vi "CRYMessage Dialog.vi"(7 "Window Title":string, 10 "YesNoCancel":T1(ring), 11 "Message Content":string) -> (2 "YesNo":bool=TRUE, 3 "Which Button?":T2(ring)=enum."Center Button")   [LabVIEW 2013]
uses:
  CRYMainGlobal.vi
panel:
  in  "Cancel Button":string
  in  "No Button":string
  in  "Yes Button":string
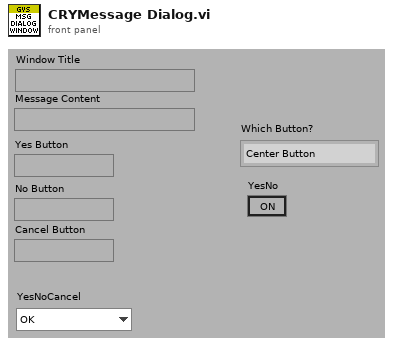
[diagram p1: front panel]
types:
  T1 = enum16{"OK", "Yes", "YesNo", "YesNoCancel", "ReplaceAppend"}
  T2 = enum16{"Left Button", "Center Button", "Right Button", "Window Close"}
  T3 = enum32{"English", "Chinese", "Korean", "Japanese", "Russian", "Chinese traditional"}
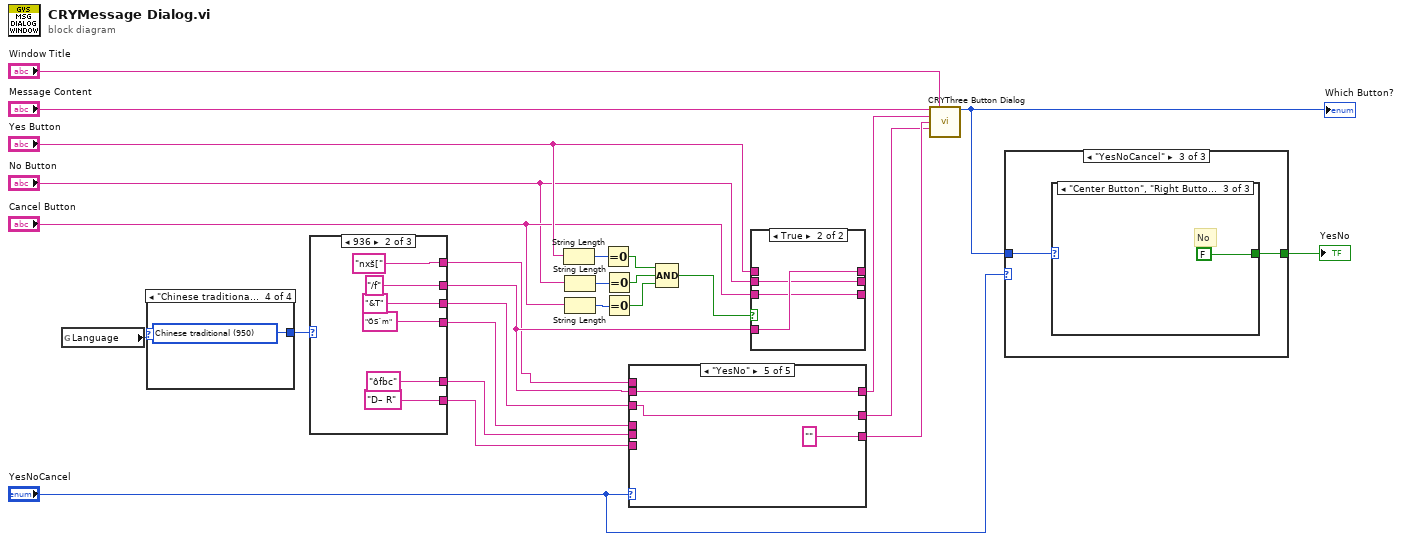
[diagram p0: block diagram]
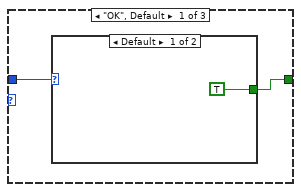
[diagram p2: hidden frame]
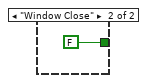
[diagram p3: hidden frame]
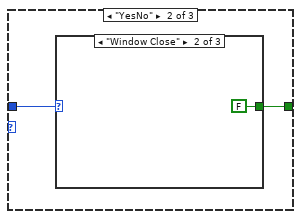
[diagram p4: hidden frame]
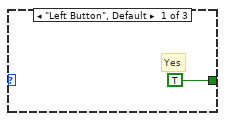
[diagram p5: hidden frame]
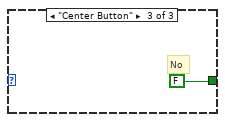
[diagram p6: hidden frame]
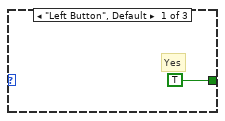
[diagram p7: hidden frame]
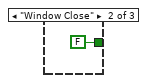
[diagram p8: hidden frame]
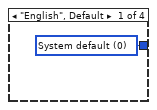
[diagram p9: hidden frame]
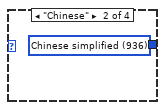
[diagram p10: hidden frame]
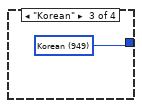
[diagram p11: hidden frame]
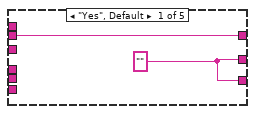
[diagram p12: hidden frame]
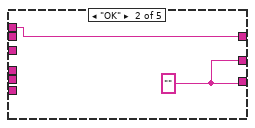
[diagram p13: hidden frame]
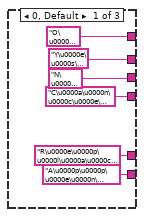
[diagram p17: hidden frame]
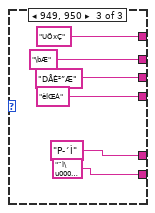
[diagram p18: hidden frame]
diagram:
  n1 = global read "CRYMainGlobal.vi" "Language"() -> (w8:T3)
  n2 = case shown="\"Chinese traditional\"" w8 {
    tunnel: [w27 w28 w29 w30] -> w7
    frame "English", Default {
      w27 = 0 items=["System default"=0, "Latin-1"=1252, "Japanese"=932, "Korean"=947, "Chinese simplified"=936, "Chinese traditional"=950, "Central Europe"=1250, "Cyrillic"=1251, "Greek"=1253, "Turkish"=1254, "Hebrew"=1255, "Arabic"=1256, "Baltic"=1257, "Thai"=874, "Vietnamese"=783, "UTF8"=65001, "UTF-7"=65000] ("Code Page")
    }
    frame "Chinese" {
      w28 = 936 items=["System default"=0, "Latin-1"=1252, "Japanese"=932, "Korean"=947, "Chinese simplified"=936, "Chinese traditional"=950, "Central Europe"=1250, "Cyrillic"=1251, "Greek"=1253, "Turkish"=1254, "Hebrew"=1255, "Arabic"=1256, "Baltic"=1257, "Thai"=874, "Vietnamese"=783, "UTF8"=65001, "UTF-7"=65000] ("Code Page")
    }
    frame "Korean" {
      w29 = 949 items=["System default"=0, "Latin-1"=1252, "Japanese"=932, "Korean"=949, "Chinese simplified"=936, "Chinese traditional"=950, "Central Europe"=1250, "Cyrillic"=1251, "Greek"=1253, "Turkish"=1254, "Hebrew"=1255, "Arabic"=1256, "Baltic"=1257, "Thai"=874, "Vietnamese"=783, "UTF8"=65001, "UTF-7"=65000] ("Code Page")
    }
    frame "Chinese traditional" {
      w30 = 950 items=["System default"=0, "Latin-1"=1252, "Japanese"=932, "Korean"=949, "Chinese simplified"=936, "Chinese traditional"=950, "Central Europe"=1250, "Cyrillic"=1251, "Greek"=1253, "Turkish"=1254, "Hebrew"=1255, "Arabic"=1256, "Baltic"=1257, "Thai"=874, "Vietnamese"=783, "UTF8"=65001, "UTF-7"=65000] ("Code Page")
    }
  }
  n3 = case shown="936" w7 {
    tunnel: ["Y\u0000e\u0000s\u0000" "/f" "\bÆ"] -> w14
    tunnel: ["N\u0000o\u0000" "&T" "DÅÈ²”Æ"] -> w13
    tunnel: ["C\u0000a\u0000n\u0000c\u0000e\u0000l\u0000" "ÖSˆm" "èÍŒÁ"] -> w12
    tunnel: ["O\u0000K\u0000" "nxš[" "UÖxÇ"] -> w6
    tunnel: ["R\u0000e\u0000p\u0000l\u0000a\u0000c\u0000e\u0000\u0000" "ôfbc" "P­´Ì"] -> w5
    tunnel: ["A\u0000p\u0000p\u0000e\u0000n\u0000d\u0000" "D– R" "¨Ì\u0000¬"] -> w4
    frame 0, Default {
    }
    frame 936 {
    }
    frame 949, 950 {
    }
  }
  n4 = String Length(string="Yes Button") -> (length=w25:i32)
  n5 = String Length(string="No Button") -> (length=w24:i32)
  n6 = String Length(string="Cancel Button") -> (length=w23:i32)
  n7 = Equal To 0?(x=w25) -> (x = 0?=w22:bool)
  n8 = Equal To 0?(x=w24) -> (x = 0?=w21:bool)
  n9 = Equal To 0?(x=w23) -> (x = 0?=w20:bool)
  n10 = case shown="\"YesNo\"" "YesNoCancel" {
    tunnel: w14 -> [w50 _ _ w58 w61]
    tunnel: w13 -> [_ _ _ w57 w60]
    tunnel: w12 -> [_ _ w53 w56 _]
    tunnel: [w50 w51 w55 w58 w61] -> w11
    tunnel: [w49 w52 w54 w57 w60] -> w9
    tunnel: [w49 w52 w53 w56 "" ("Yes Button")] -> w10
    tunnel: w6 -> [_ w51 _ _ _]
    tunnel: w5 -> [_ _ w55 _ _]
    tunnel: w4 -> [_ _ w54 _ _]
    frame "Yes", Default {
      w49 = "" ("Yes Button")
    }
    frame "OK" {
      w52 = "" ("Yes Button")
    }
    frame "ReplaceAppend" {
    }
    frame "YesNoCancel" {
    }
    frame "YesNo" {
    }
  }
  n11 = Compound Arithmetic op=AND(w22, w21, w20) -> (w19:bool)
  n12 = case shown="True" w19 {
    tunnel: w14 -> [_ w67]
    tunnel: "Yes Button" -> [w64 _]
    tunnel: "Cancel Button" -> [w62 w65]
    tunnel: "No Button" -> [w63 w66]
    tunnel: [w64 w67] -> _
    tunnel: [w63 w66] -> _
    tunnel: [w62 w65] -> _
    frame False {
    }
    frame True {
    }
  }
  n13 = call "CRYThree Button Dialog.vi"("message"="Message Content", "Window Title (\"\")"="Window Title", "Left Button Text (\"Yes\")"=w11, "Right Button Text (\"Cancel\")"=w10, "Center Button Text (\"No\")"=w9) -> ("Which Button?"=w2:T2)  [unwired: 10 in]
  "Which Button?" <- w2
  n14 = case shown="\"YesNoCancel\"" "YesNoCancel" {
    tunnel: w2 -> [w68 w73 w78]
    tunnel: [w69 w72 w77] -> w1
    frame "OK", Default {
      n15 = case shown="Default" w68 {
        tunnel: [TRUE FALSE] -> w69
        frame Default {
        }
        frame "Window Close" {
        }
      }
    }
    frame "YesNo" {
      n16 = case shown="\"Window Close\"" w73 {
        tunnel: [TRUE FALSE FALSE] -> w72
        frame "Left Button", Default {
          # "Yes"
        }
        frame "Window Close" {
        }
        frame "Center Button" {
          # "No"
        }
      }
    }
    frame "YesNoCancel" {
      n17 = case shown="\"Center Button\", \"Right Button\"" w78 {
        tunnel: [TRUE FALSE FALSE] -> w77
        frame "Left Button", Default {
          # "Yes"
        }
        frame "Window Close" {
        }
        frame "Center Button", "Right Button" {
          # "No"
        }
      }
    }
  }
  "YesNo" <- w1
